vi "Test shm get Event summary State LV.vi"(8 "error in (no error)":errorcluster, 11 "logevent_summaryState_Ctl":cluster{"summaryState":i32, "priority":i32}) -> (0 "error out":errorcluster, 2 "function return":i32, 3 "logevent_summaryState_Ctl out":cluster{"summaryState":i32, "priority":i32})   [LabVIEW 2018, in "SALLV_Test.lvlib"]
doc: "int Test_shm_getEvent_summaryStateLV(Test_logevent_summaryStateLV *logevent_summaryState_Ctl );"
uses:
  SALLV_Test.lvlib
  SALLV_Test.so
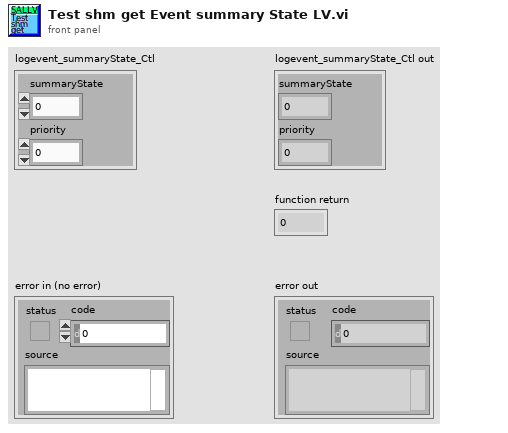
[diagram p1: front panel]
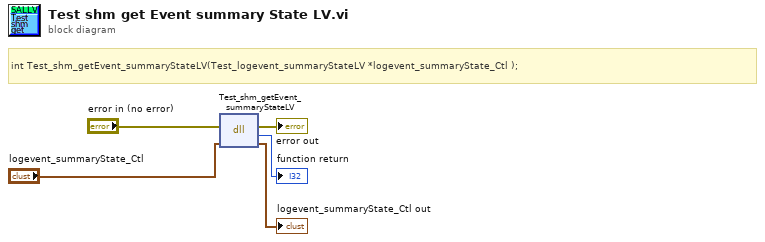
[diagram p0: block diagram]
diagram:
  # "int Test_shm_getEvent_summaryStateLV(Test_logevent_summaryStateLV *logevent_summaryState_Ctl );"
  n1 = dll-call lib="home/ttsai/Documents/salLabVIEWtestData/SALLV_Test.*" fn="Test_shm_getEvent_summaryStateLV"(error in="error in (no error)", "logevent_summaryState_Ctl"="logevent_summaryState_Ctl") -> (error out=→"error out":errorcluster, →"function return":i32, "logevent_summaryState_Ctl"=→"logevent_summaryState_Ctl out":cluster{"summaryState":i32, "priority":i32})  [unwired: 2 in, 1 out]
